vi "KeyInCounterPosition V0.41.vi"() -> (1 "Counter Position output":dbl=950.0 min=0.0 max=2600.0 format="%.3f", 2 "Stepper Position":i32)   [LabVIEW 2019]
panel:
  in  "?":bool
  in  "Counter Position":dbl=7000.0 min=0.0 max=26000.0 format="%.3f"
  # "Please input your own counter position,\nand then click \"OK\" button."
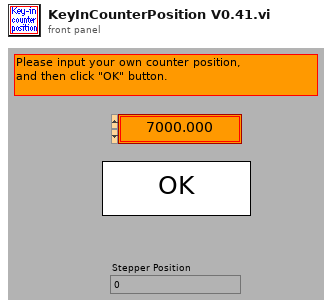
[diagram p1: front panel]
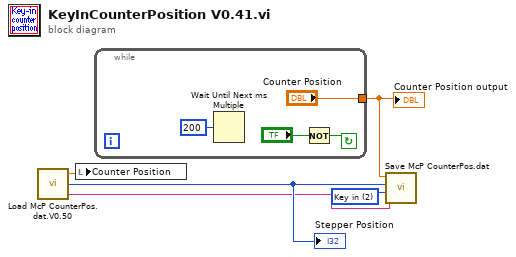
[diagram p0: block diagram]
diagram:
  w1 = u16 2 items=["Moving", "Calibration", "Key in", "Initialization"] ("Set Method")
  n1 = call "Load McP CounterPos.dat.V0.50.vi"() -> ("Counter Position"=w2:dbl, "Stepper Position"=w5:i32, "Last Calibration Date"=w4:string)  [unwired: 1 in]
  "Stepper Position" <- w5
  n2 = local write "Counter Position"(w2) -> ()
  n3 = while {
    tunnel: ["Counter Position"] -> w3
    stop <- w9 continue-if-true
    n4 = Wait Until Next ms Multiple(millisecond multiple=u32 200) -> ()  [unwired: 1 out]
    n5 = Not(x="?") -> (.not. x?=w9:bool)
  }
  "Counter Position output" <- w3
  n6 = call "Save McP CounterPos.dat.vi"("Last Calibration Date"=w4, "Set Method"=w1, "McP Stepper Position"=w5, "McP Counter Position"=w3) -> ()  [unwired: 2 in, 1 out]
